vi "Twitter Open - Embedded.vi"(5 "Access Secret":string, 7 "Access Token":string, 8 "error in":errorcluster, 10 "Consumer Secret":string, 11 "Consumer Key":string) -> (0 "error out":errorcluster, 3 "Twitter Handle Out":T1={"OAuth Credentials"={"Signature Method"=enum."HMAC-SHA1", "Version"="1.0", "Client"={"Token"="", "Secret"=""}, "Access"={"Token"="", "Secret"=""}}, "since ID"="", "max ID"="", "Screen Name"=""})   [LabVIEW 2011, in "i3-twitter.lvlib"]
doc: "<b>Twitter Open - Embedded</b> is used when the application has a specific set of Access Credentials or the user is on a platform without a web browser.\n\nThe <b>Consumer Key</b> and <b>Consumer Secret</b> are unique to each application and can be created by making an application at dev.twitter.com. For more information and a Getting Started tutorial navigate to Help » i3 Twitter Help in LabVIEW.\n\nUse of this function requires <b>Access Credentials</b> which can be found on dev.twitter.com when an application is created or by using the <b>Twitter Open - Desktop VI</b> on a computer with a Web Browser to have the user grant access and create an Access Token and Access Secret for use on the embedded system."
uses:
  i3-twitter.lvlib
  Controls/Twitter Handle.ctl
  i3-oauth/Controls/OAuth Handle.ctl
  i3-oauth/Controls/Signature Method.ctl
  i3-oauth/Controls/Credentials.ctl
  <vilib>/Utility/error.llb/whitespace.ctl
  i3-oauth/i3-oauth.lvlib
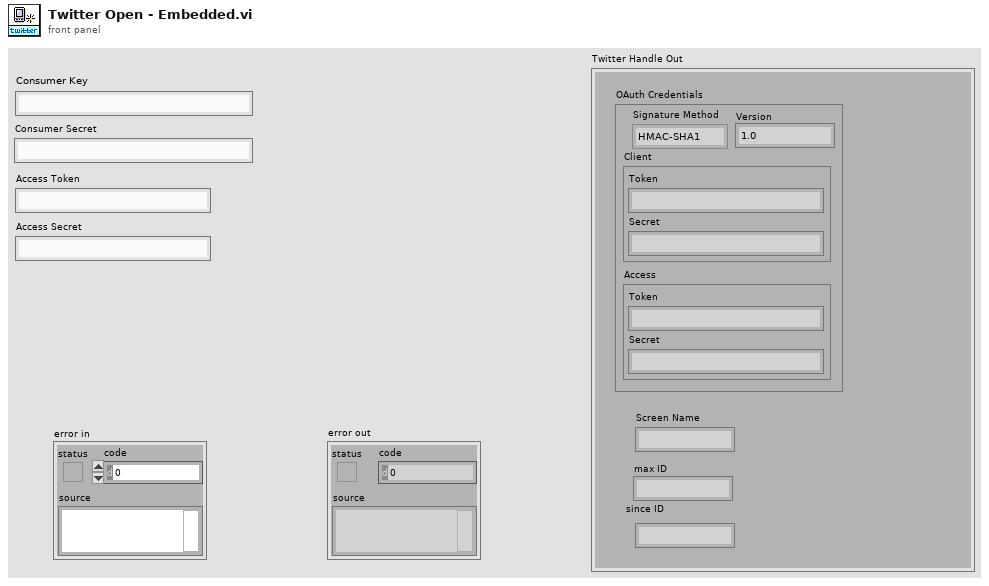
[diagram p1: front panel]
types:
  T1 = typedef "i3-twitter.lvlib/Twitter Handle.ctl" = cluster{"OAuth Credentials":T2, "since ID":string, "max ID":string, "Screen Name":string}
  T2 = typedef "i3-oauth.lvlib/OAuth Handle.ctl" = cluster{"Signature Method":T3, "Version":string, "Client":T4, "Access":T4}
  T3 = typedef "i3-oauth.lvlib/Signature Method.ctl" = enum16{"HMAC-MD5", "HMAC-SHA1", "HMAC-SHA224", "HMAC-SHA256", "HMAC-SHA384", "HMAC-SHA512"}
  T4 = typedef "i3-oauth.lvlib/Credentials.ctl" = cluster{"Token":string, "Secret":string}
  T5 = typedef "whitespace.ctl" = u16
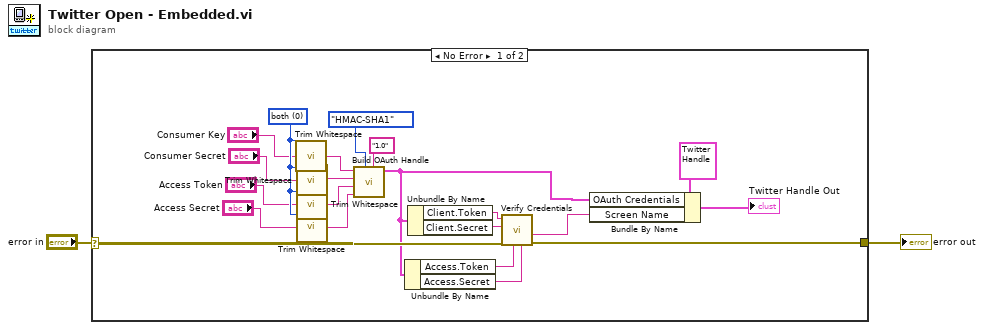
[diagram p0: block diagram]
diagram:
  n1 = case shown="No Error" "error in" {
    selector: "error in" -> [w18 w24]
    tunnel: [w21 w24] -> w2
    frame No Error {
      w23 = T5 0 items=["both", "start of string", "end of string"] ("location (both)")
      n2 = call <vilib>:"Trim Whitespace.vi"("string"="Consumer Key", "location (both)"=w23) -> ("trimmed string"=w9:string)
      n3 = call <vilib>:"Trim Whitespace.vi"("string"="Consumer Secret", "location (both)"=w23) -> ("trimmed string"=w8:string)
      n4 = call <vilib>:"Trim Whitespace.vi"("string"="Access Token", "location (both)"=w23) -> ("trimmed string"=w7:string)
      n5 = call <vilib>:"Trim Whitespace.vi"("string"="Access Secret", "location (both)"=w23) -> ("trimmed string"=w6:string)
      n6 = call "Build OAuth Handle.vi"("Version (1.0)"="1.0", "Signature Method (HMAC-SHA1)"=Signature_Method."HMAC-SHA1", "Access Secret"=w6, "Access Token"=w7, "Client Secret"=w8, "Client Token"=w9) -> ("OAuth Handle"=w11:T2)  [unwired: 5 in]
      n7 = Unbundle By Name(w11) -> ("Access.Token"=w13:string, "Access.Secret"=w12:string)
      n8 = Unbundle By Name(w11) -> ("Client.Token"=w14:string, "Client.Secret"=w15:string)
      n9 = call "Verify Credentials.vi"("Access Token Secret (In)"=w12, "Access Token (In)"=w13, "error in (no error)"=w18, "Consumer Secret"=w15, "Consumer Key"=w14) -> ("error out"=w21:errorcluster, "Screen Name"=w20:string)  [unwired: 3 in, 2 out]
      n10 = Bundle By Name(cluster=T1 {"OAuth Credentials"={"Signature Method"=enum."HMAC-MD5", "Version"="", "Client"={"Token"="", "Secret"=""}, "Access"={"Token"="", "Secret"=""}}, "since ID"="", "max ID"="", "Screen Name"=""} ("Twitter Handle"), "OAuth Credentials"=w11, "Screen Name"=w20) -> (→"Twitter Handle Out":T1)
    }
    frame Error {
    }
  }
  "error out" <- w2
